vi "Decode I32.vi"(10 "Pixel Offset (0)":i32, 11 "Image In":u8[](array[numeric])) -> (3 "I32":i32)   [LabVIEW 2020]
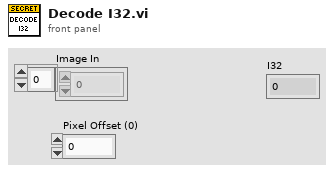
[diagram p1: front panel]
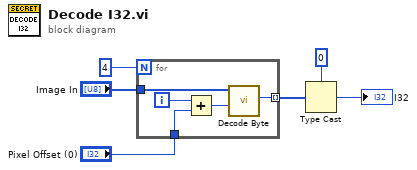
[diagram p0: block diagram]
diagram:
  n1 = for {
    N: 4 -> [_]
    tunnel: "Image In" -> [w11]
    tunnel: [w9] -> w5 mode=indexing
    tunnel: "Pixel Offset (0)" -> [w7]
    i -> [w10]
    n2 = Add(x=w10, y=w7) -> (x+y=w8:i32)
    n3 = call "Decode Byte.vi"("Pixel Offset"=w8, "Image In"=w11) -> ("Decoded Byte"=w9:u8)  [unwired: 9 in]
  }
  n4 = Type Cast(type=0, x=w5) -> (*(type *) &x=→"I32":i32)
